vi "CheckLimits.vi"(8 "error in (no error)":errorcluster, 9 "Lower Limit":dbl[](array[numeric]), 10 "Upper Limit":dbl[](array[numeric]), 11 "Signal":dbl[](array[numeric])) -> (0 "error out":errorcluster, 1 "Passed?":i32, 2 "Status":string, 3 "Overall test passed?":bool)   [LabVIEW 2021]
uses:
  <vilib>/measure/NI_MAPro.lvlib
panel:
  out "Waveform Chart":dbl[][](graph)
  out "Individual test results":bool[](array[boolean])
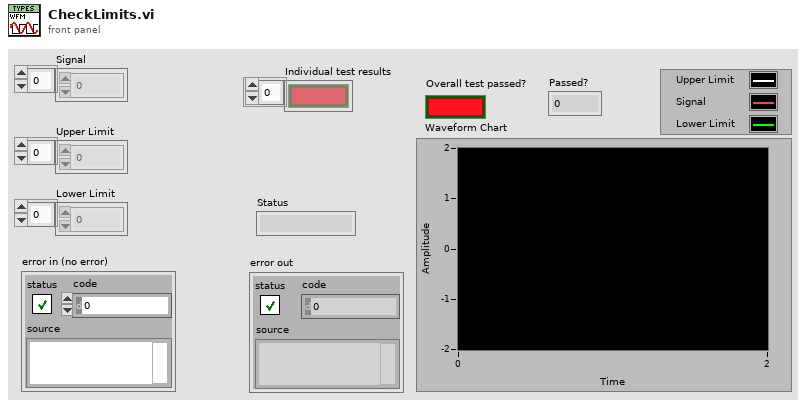
[diagram p1: front panel]
types:
  T1 = cluster{"pass region":i32, "include UL":bool, "include LL":bool}
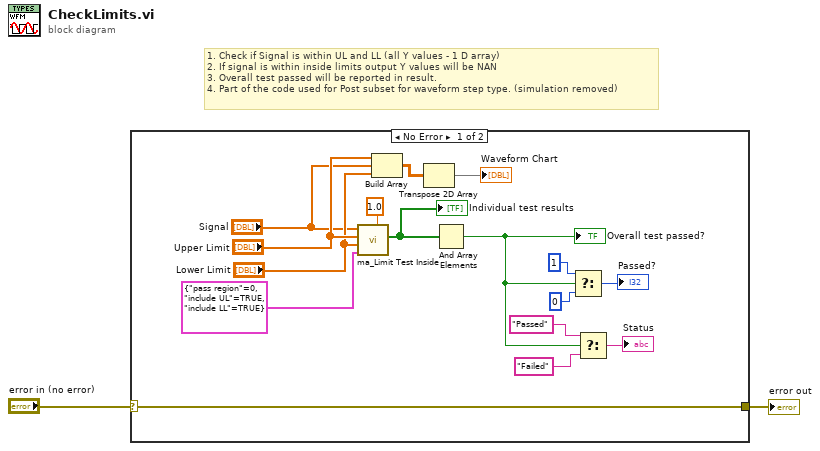
[diagram p0: block diagram]
diagram:
  # "1. Check if Signal is within UL and LL (all Y values - 1 D array)\n2. If signal is within inside limits output Y values will be NAN\n3. Overall test passed will be reported in result.\n4. Part of the code used for Post subset for waveform step type. (simulation removed)"
  n1 = case shown="No Error" "error in (no error)" {
    selector: "error in (no error)" -> [w3 w19]
    tunnel: [w3 w19] -> w1
    frame No Error {
      n2 = call <vilib>:"ma_Limit Test Inside.vi"("x0"=1.0, "limit test config"=T1 {"pass region"=0, "include UL"=TRUE, "include LL"=TRUE}, "lower"="Lower Limit", "upper"="Upper Limit", "signal"="Signal") -> ("test results"=w18:bool[])  [unwired: 1 in, 5 out]
      "Individual test results" <- w18
      n3 = Build Array("Upper Limit", "Signal", "Lower Limit") -> (w15:dbl[][])
      n4 = Transpose 2D Array(2D array=w15) -> (transposed array=→"Waveform Chart":dbl[][])
      n5 = And Array Elements(Boolean array=w18) -> (logical AND=w7:bool)
      "Overall test passed?" <- w7
      n6 = Select(t=1, s=w7, f=0) -> (s? t:f=→"Passed?":i32)
      n7 = Select(t="Passed", s=w7, f="Failed") -> (s? t:f=→"Status":string)
    }
    frame Error {
    }
  }
  "error out" <- w1
